vi "大气压力盐度设置.vi"(8 "error in (no error)":errorcluster caption="错误输入（无错误）", 10 "盐度":sgl, 11 "大气压力":sgl) -> (0 "error out":errorcluster caption="错误输出")   [LabVIEW 2016, in "NAQ_DO.lvlib"]
uses:
  NAQ_DO.lvlib
  <vilib>/Plasmionique/MB Master/MB_Master_Serial/MB_Master_Serial.lvclass
  C:/Program Files (x86)/National Instruments/LabVIEW 2016/vi.lib/Plasmionique/MB Master/MB_Master/MB_Master.lvclass
  <vilib>/Plasmionique/MB Master/MB Master.lvlib
  DAM395CF/PLC.lvlib
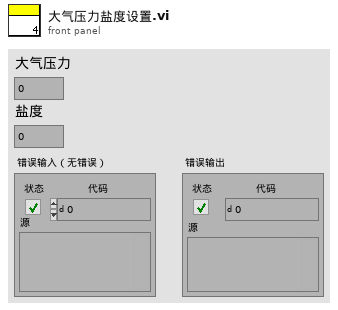
[diagram p1: front panel]
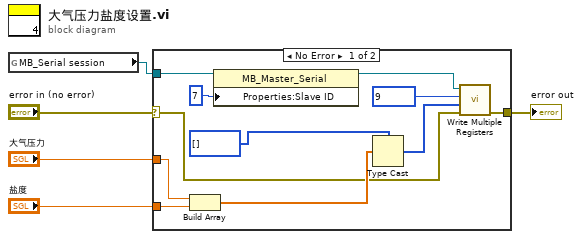
[diagram p0: block diagram]
diagram:
  n1 = global read "中间变量.vi" "MB_Serial session"() -> (w1:refnum<class "MB_Master_Serial.lvclass">)
  n2 = case shown="No Error" "error in (no error)" {
    selector: "error in (no error)" -> [w10 w17]
    tunnel: [w16 w17] -> w5
    tunnel: w1 -> [w9 _]
    tunnel: "大气压力" -> [w8 _]
    tunnel: "盐度" -> [w7 _]
    frame No Error {
      n3 = Build Array(w8, w7) -> (w11:sgl[])
      n4 = property class="MB_Master_Serial"(reference=w9, "Properties:Slave ID"=7) -> (reference out=w14:refnum<class "MB_Master_Serial.lvclass">)  [unwired: 1 in, 1 out]
      n5 = Type Cast(type=u16[] [], x=w11) -> (*(type *) &x=w6:u16[])
      n6 = call <vilib>:"Write Multiple Registers.vi"("error in (no error)"=w10, "values"=w6, "starting address"=u16 9, "MB session in"=w14) -> ("error out"=w16:errorcluster)  [unwired: 6 in, 1 out]
    }
    frame Error {
    }
  }
  "error out" <- w5
